vi "Get Array of Points to Measure.vi"(8 "error in":errorcluster, 11 "eye scan in":refnum<class "niHighSpeedSerial N Point Eye Scan v1 Host.lvclass">) -> (0 "error out":errorcluster, 2 "array of points to measure":T1[](array[typedef]), 3 "eye scan out":refnum<class "niHighSpeedSerial N Point Eye Scan v1 Host.lvclass">)   [LabVIEW 2014, in "niHighSpeedSerial N Point Eye Scan v1 Host.lvclass"]
doc: "Returns the array of point offsets that were requested to be measured.\n\n<B>Input Parameters</B>\n\n<B>error in</B> describes error conditions that occur before this node runs. This input provides standard 'error in' functionality.\n\n<B>eye scan in</B> Takes in a reference to your session from the previous VI.\n\n<B>Output Parameters</B>\n\n<B>error out</B> contains error information. This output provides standard 'error out' functionality.\n\n<B>array of points to measure</B> is the array of point offsets to measure using Eye Scan.\n\n<B>array of points to measure.horizontal offset</B> is the horizontal offset of the point to measure.\n\n<B>array of points to measure.vertical offset</B> is the vertical offset of the point to measure.\n\n<B>eye scan out</B> passes a reference to your session to the next VI."
uses:
  <instrlib>/niHighSpeedSerial/Eye Scan/v1/Host/Impl/N Point Eye Scan/niHighSpeedSerial N Point Eye Scan v1 Host.lvclass
  <instrlib>/niHighSpeedSerial/Eye Scan/v1/Host/Common/Public/Point Offsets.ctl
  <instrlib>/niHighSpeedSerial/Eye Scan/v1/Host/Impl/N Point Eye Scan/niHighSpeedSerial N Point Eye Scan v1 Host.lvclass/niHighSpeedSerial N Point Eye Scan v1 Host.ctl
  <instrlib>/niHighSpeedSerial/Eye Scan/v1/Host/Common/niHighSpeedSerial Eye Scan Common v1 Host.lvlib
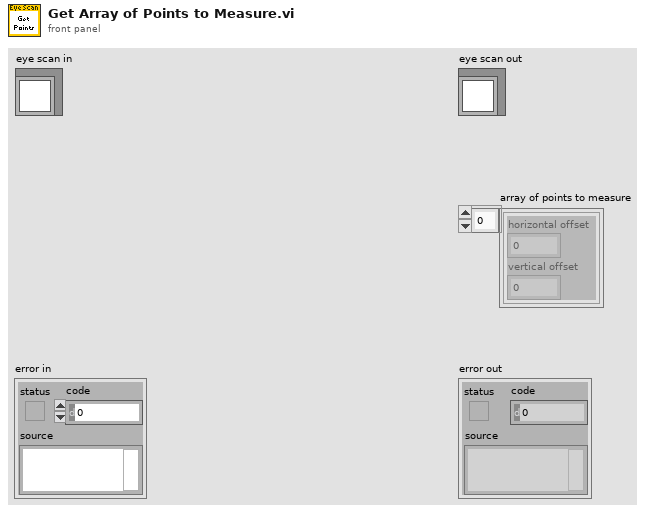
[diagram p1: front panel]
types:
  T1 = typedef "niHighSpeedSerial Eye Scan Common v1 Host.lvlib/Point Offsets.ctl" = cluster{"horizontal offset":i16, "vertical offset":i8}
  T2 = typedef "N Point Eye Scan v1 Host.lvclass/Private Data.ctl" = cluster{"array of points to measure":T1[], "n point eye scan point iterator":refnum<class "niHighSpeedSerial N Point Eye Scan Point Iterator v1 Host.lvclass">}
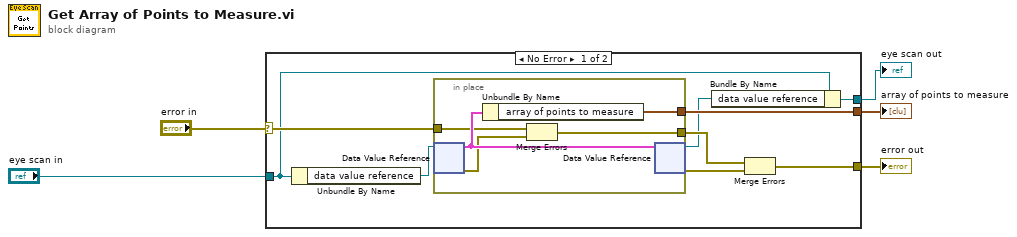
[diagram p0: block diagram]
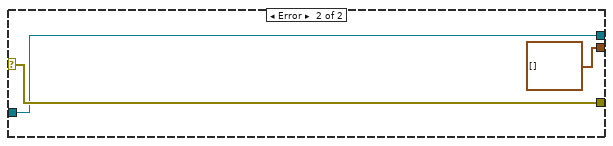
[diagram p2: hidden frame]
diagram:
  n1 = case shown="No Error" "error in" {
    selector: "error in" -> [w12 w22]
    tunnel: [w9 w22] -> w4
    tunnel: [w7 w21] -> w2
    tunnel: "eye scan in" -> [w8 w21]
    tunnel: [w13 T1[] [] ("array of points to measure")] -> w1
    frame No Error {
      n2 = Unbundle By Name(w8) -> ("data value reference"=w14:refnum<data-value>)
      n3 = in-place {
        in-place-border: [w19] -> w13
        in-place-border: w12 -> [w17]
        in-place-border: [w15] -> w10
        n4 = in-place-dvr #1(w14) -> (w18:T2, w16:errorcluster)
        n5 = Unbundle By Name(w18) -> ("array of points to measure"=w19:T1[])
        n6 = Merge Errors(w17, w16) -> (w15:errorcluster)
        n7 = in-place-dvr #1(w18) -> (w6:refnum<data-value>, w11:errorcluster)
      }
      n8 = Bundle By Name(cluster=w8, "data value reference"=w6) -> (w7:refnum<class "niHighSpeedSerial N Point Eye Scan v1 Host.lvclass">)
      n9 = Merge Errors(w10, w11) -> (w9:errorcluster)
    }
    frame Error {
    }
  }
  "error out" <- w4
  "eye scan out" <- w2
  "array of points to measure" <- w1
